vi "SocketHook.vi"(0 "Socket in":refnum<class "Socket.lvclass">, 2 "Mode":T1(ring), 7 "data in":string, 11 "error in (no error)":errorcluster) -> (4 "Socket out":refnum<class "Socket.lvclass">, 8 "data out":string, 15 "error out":errorcluster)   [LabVIEW 2011, in "Socket.lvclass"]
uses:
  Socket.lvclass
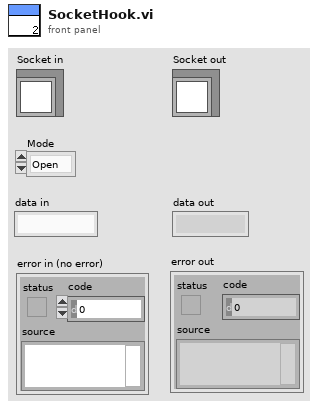
[diagram p1: front panel]
types:
  T1 = enum16{"Open", "R", "W", "R->W", "W->R", "Close"}
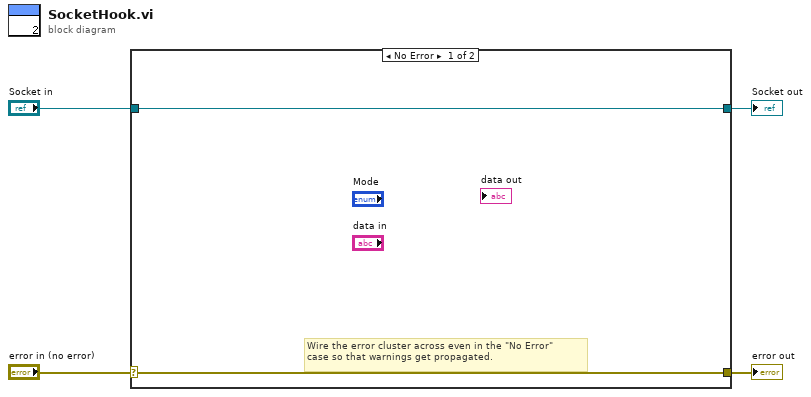
[diagram p0: block diagram]
diagram:
  n1 = case shown="No Error" "error in (no error)" {
    selector: "error in (no error)" -> [w5 w8]
    tunnel: [w5 w8] -> w3
    tunnel: [w6 w7] -> w1
    tunnel: "Socket in" -> [w6 w7]
    frame No Error {
      # "Wire the error cluster across even in the \"No Error\"\ncase so that warnings get propagated."
    }
    frame Error {
    }
  }
  "error out" <- w3
  "Socket out" <- w1
